vi "List Output.vi"(0 "VISA resource name":refnum<visa-resource-name>, 1 "Serial Configuration":T2={"Baud Rate"=9600, "Parity"=0, "Data Bits"=8, "Stop Bits"=10, "Flow Control"=0} {"Flow Control" items=["None", "XON/XOFF", "RTS/CTS", "XON/XOFF & RTS/CTS", "DTR/DSR", "XON/XOFF & DTR/DSR"]; "Stop Bits" items=["1.0"=10, "1.5"=15, "2.0"=20]; "Data Bits" items=["7"=7, "8"=8]; "Parity" items=["None", "Odd", "Even", "Mark", "Space"]; "Baud Rate" items=["300"=300, "600"=600, "1200"=1200, "2400"=2400, "4800"=4800, "9600"=9600, "19200"=19200, "38400"=38400, "57600"=57600, "115200"=115200]}, 2 "Supply Settings":T1={"Repeat"=0, "Terminate Type"=0, "Save File"=1, "Type"=0, "Normal Current(A)"=0.0, "Normal Voltage(V)"=0.0} {"Normal Voltage(V)" min=0.0; "Type" items=["Current", "Voltage"]; "Save File" min=1 max=10; "Terminate Type" items=["Normal", "Last", "Off"]; "Repeat" min=0}, 5 "error in":errorcluster, 6 "Level(V/A/W/ohm)":dbl[](array[numeric]) min=0.0, 8 "Dwell(S)":dbl[](array[numeric]) min=0.0, 10 "Slew":dbl[](array[numeric]) min=0.0) -> (14 "VISA resource name out":refnum<visa-resource-name>, 19 "error out":errorcluster)   [LabVIEW 2025, in "IT-M3900C.lvlib"]
doc: "This example is used to edit the user - defined waveform function in source mode, call and implement the waveform output."
uses:
  IT-M3900C.lvlib
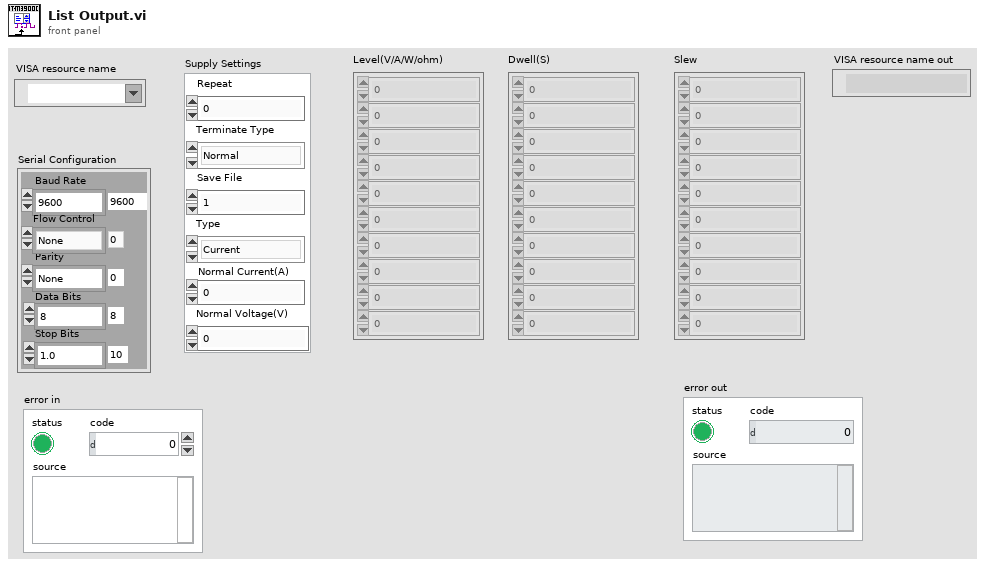
[diagram p1: front panel]
types:
  T1 = cluster{"Repeat":i32, "Terminate Type":u16, "Save File":i32, "Type":u16, "Normal Current(A)":dbl, "Normal Voltage(V)":dbl}
  T2 = cluster{"Baud Rate":u32, "Parity":u16, "Data Bits":u16, "Stop Bits":u16, "Flow Control":u16}
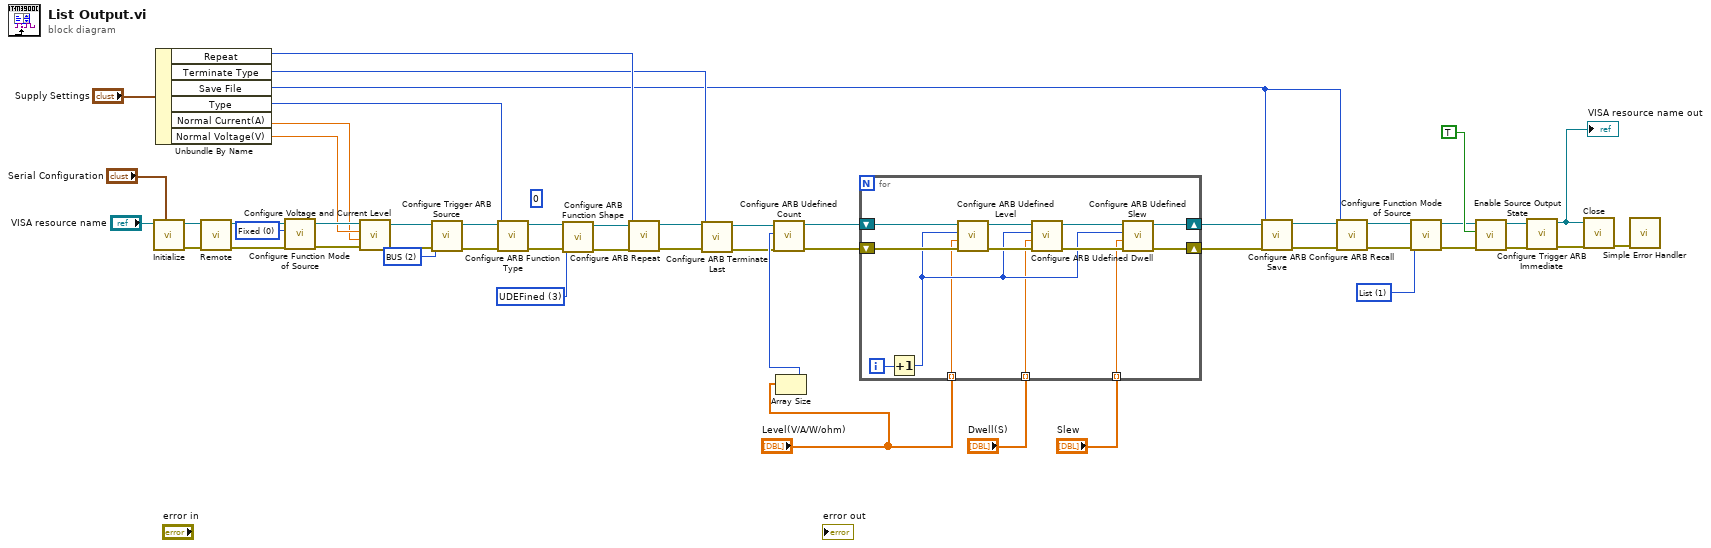
[diagram p0: block diagram]
diagram:
  (unwired) u16 0 ("Type")
  w14 = u16 0 items=["Fixed", "List", "Battery", "Solar", "CarProfile", "Fuel", "Step"] ("Mode")
  w19 = u16 1 items=["Fixed", "List", "Battery", "Solar", "CarProfile", "Fuel", "Step"] ("Mode")
  w25 = u16 2 items=["IMMediate", "MANual", "BUS", "EXTernal"] ("Source")
  w39 = u16 3 items=["PULSe", "SINusiod", "SWEepsine", "UDEFined", "CDWell", "SEQuence"] ("Type")
  n1 = call "Initialize.vi"("Serial Configuration"="Serial Configuration", "VISA resource name"="VISA resource name") -> ("error out"=w48:errorcluster, "VISA resource name out"=w49:refnum<visa-resource-name>)  [unwired: 8 in]
  n2 = Unbundle By Name("Supply Settings") -> ("Repeat"=w4:i32, "Terminate Type"=w3:u16, "Save File"=w1:i32, "Type"=w2:u16, "Normal Current(A)"=w5:dbl, "Normal Voltage(V)"=w6:dbl)
  n3 = call "Remote.vi"("error in"=w48, "VISA resource name"=w49) -> ("error out"=w17:errorcluster, "VISA resource name out"=w18:refnum<visa-resource-name>)  [unwired: 8 in]
  n4 = call "Configure Function Mode of Source.vi"("error in"=w17, "Mode"=w14, "VISA resource name"=w18) -> ("error out"=w16:errorcluster, "VISA resource name out"=w15:refnum<visa-resource-name>)  [unwired: 7 in]
  n5 = call "Configure Voltage and Current Level.vi"("error in"=w16, "Current(A)"=w5, "Voltage(V)"=w6, "VISA resource name"=w15) -> ("error out"=w21:errorcluster, "VISA resource name out"=w20:refnum<visa-resource-name>)  [unwired: 6 in]
  n6 = call "Configure Trigger ARB Source.vi"("error in"=w21, "Source"=w25, "VISA resource name"=w20) -> ("error out"=w27:errorcluster, "VISA resource name out"=w26:refnum<visa-resource-name>)  [unwired: 7 in]
  n7 = call "Configure ARB Function Type.vi"("error in"=w27, "Type"=w2, "VISA resource name"=w26) -> ("error out"=w40:errorcluster, "VISA resource name out"=w41:refnum<visa-resource-name>)  [unwired: 7 in]
  n8 = call "Configure ARB Function Shape.vi"("error in"=w40, "Type"=w39, "VISA resource name"=w41) -> ("error out"=w37:errorcluster, "VISA resource name out"=w38:refnum<visa-resource-name>)  [unwired: 7 in]
  n9 = call "Configure ARB Repeat.vi"("error in"=w37, "Repeat"=w4, "VISA resource name"=w38) -> ("error out"=w35:errorcluster, "VISA resource name out"=w36:refnum<visa-resource-name>)  [unwired: 7 in]
  n10 = call "Configure ARB Terminate Last.vi"("error in"=w35, "Type"=w3, "VISA resource name"=w36) -> ("error out"=w33:errorcluster, "VISA resource name out"=w34:refnum<visa-resource-name>)  [unwired: 7 in]
  n11 = Array Size(array="Level(V/A/W/ohm)") -> (size(s)=w44:i32)
  n12 = call "Configure ARB Udefined Count.vi"("error in"=w33, "Count"=w44, "VISA resource name"=w34) -> ("error out"=w46:errorcluster, "VISA resource name out"=w47:refnum<visa-resource-name>)  [unwired: 7 in]
  n13 = for {
    shift-right: [w58] -> w32
    shift-left: w47 -> [w64]
    shift-right: [w57] -> w31
    shift-left: w46 -> [w63]
    tunnel: "Level(V/A/W/ohm)" -> [w54] mode=indexing
    tunnel: "Dwell(S)" -> [w53] mode=indexing
    tunnel: "Slew" -> [w52] mode=indexing
    i -> [w56]
    n14 = Increment(x=w56) -> (x+1=w55:i32)
    n15 = call "Configure ARB Udefined Level.vi"("error in"=w63, "Level"=w54, "Step"=w55, "VISA resource name"=w64) -> ("error out"=w61:errorcluster, "VISA resource name out"=w62:refnum<visa-resource-name>)  [unwired: 6 in]
    n16 = call "Configure ARB Udefined Dwell.vi"("error in"=w61, "DWELl"=w53, "Step"=w55, "VISA resource name"=w62) -> ("error out"=w59:errorcluster, "VISA resource name out"=w60:refnum<visa-resource-name>)  [unwired: 6 in]
    n17 = call "Configure ARB Udefined Slew.vi"("error in"=w59, "Slew"=w52, "Step"=w55, "VISA resource name"=w60) -> ("error out"=w57:errorcluster, "VISA resource name out"=w58:refnum<visa-resource-name>)  [unwired: 6 in]
  }
  n18 = call "Configure ARB Save.vi"("error in"=w31, "File"=w1, "VISA resource name"=w32) -> ("error out"=w30:errorcluster, "VISA resource name out"=w29:refnum<visa-resource-name>)  [unwired: 7 in]
  n19 = call "Configure ARB Recall.vi"("error in"=w30, "File"=w1, "VISA resource name"=w29) -> ("error out"=w12:errorcluster, "VISA resource name out"=w13:refnum<visa-resource-name>)  [unwired: 7 in]
  n20 = call "Configure Function Mode of Source.vi"("error in"=w12, "Mode"=w19, "VISA resource name"=w13) -> ("error out"=w10:errorcluster, "VISA resource name out"=w11:refnum<visa-resource-name>)  [unwired: 7 in]
  n21 = call "Enable Source Output State.vi"("error in"=w10, "State"=TRUE, "VISA resource name"=w11) -> ("error out"=w9:errorcluster, "VISA resource name out"=w8:refnum<visa-resource-name>)  [unwired: 7 in]
  n22 = call "Configure Trigger ARB Immediate.vi"("error in"=w9, "VISA resource name"=w8) -> ("error out"=w23:errorcluster, "VISA resource name out"=w24:refnum<visa-resource-name>)  [unwired: 8 in]
  "VISA resource name out" <- w24
  n23 = call "Close.vi"("error in"=w23, "VISA resource name"=w24) -> ("error out"=w50:errorcluster)  [unwired: 9 in]
  n24 = call <vilib>:"Simple Error Handler.vi"("error in (no error)"=w50) -> ()  [unwired: 4 in, 5 out]
